vi "Approach then IT.vi"(7 "Computer called (T/F)":bool) -> ()   [LabVIEW 2023]
uses:
  Sub_Vi/TypeDefsControls/Zposition.ctl
  Sub_Vi/TypeDefsControls/Piezo Velocity.ctl
  Sub_Vi/TypeDefsControls/Voltage.ctl
  Sub_Vi/TypeDefsControls/Xposition.ctl
  Sub_Vi/TypeDefsControls/Yposition.ctl
  Sub_Vi/TypeDefsControls/Time.ctl
  Sub_Vi/TypeDefs/WayPointCluster.ctl
  Sub_Vi/TypeDefs/ChangeOnFly.ctl
  Sub_Vi/TypeDefs/Display.ctl
  Sub_Vi/TypeDefs/Settings.ctl
  Sub_Vi/TypeDefsControls/Feedback Type.ctl
  Settings.vi
panel:
  in  "Tab Control 2":T1(tab)
  out "C1":dbl[](graph)
  out "C2":dbl[](graph)
  out "C3":dbl[](graph)
  in  "Feedback Type":T2=enum."Current 1"
  in  "Tab Control":enum32{"C1 vs Z", "C2 vs Z", "C3 vs Z"}(tab)
  out "Z vs C1":cluster{"Y":dbl[], "Y":dbl[]}[](graph)
  out "Z vs C2":cluster{"Y":dbl[], "Y":dbl[]}[](graph)
  out "Z vs C3":cluster{"Y":dbl[], "Y":dbl[]}[](graph)
  in  "SettingsCluster":T3={"Sample Rate (us)"=1, "Samples Per Data Point (int, power of 2)"=1000, "DistanceToBulk (um)"=-1.0, "HoldTimeScaler"=1, "SaveData"=TRUE, "DistanceToBulk (um) 2"=-1.0, "DistanceToBulk (um) 3"=-1.0}
  in  "Display Cluster":T4
  in  "ChangeonFly":T5
  in  "WayPointCluster":T6
  in  "IT Time (s)":T7=8.0 min=0.0
  in  "Start scan Button":bool
  in  "Stop":bool
  in  "Pause":bool
  in  "IT Voltage (V)":T8 min=-10.0 max=10.0
  in  "Greater Than":bool=TRUE
  in  "Set X":bool
  in  "Set Y":bool
  in  "Y":T9=50.0 min=0.0 max=100000.0
  in  "X":T10=50.0 min=0.0 max=100000.0
  in  "Retract after approach":bool=TRUE
  in  "Approach Voltage (V)":T8=0.35 min=-10.0 max=10.0
  in  "Approach Rate (µm/s)":T11=0.1 min=0.0
  in  "End Extension (µm)":T12 min=0.0 max=100000.0
  in  "Start Extention (µm)":T12=150.0 min=0.0 max=100000.0
  in  "Feedback Threshold (A)":dbl
  in  "Start Scanning Button":bool
  out "Lockin Phase":dbl[](graph)
  out "Lockin Amp":dbl[](graph)
  # "Settings"
  # "Pause at"
  # "Advanced Settings"
  # "IT Controls"
  # "Voltage Profile"
  # "Approach"
  # "Retract"
  # "IT"
  # "IT\nVoltage"
  # "Approach\nVoltage"
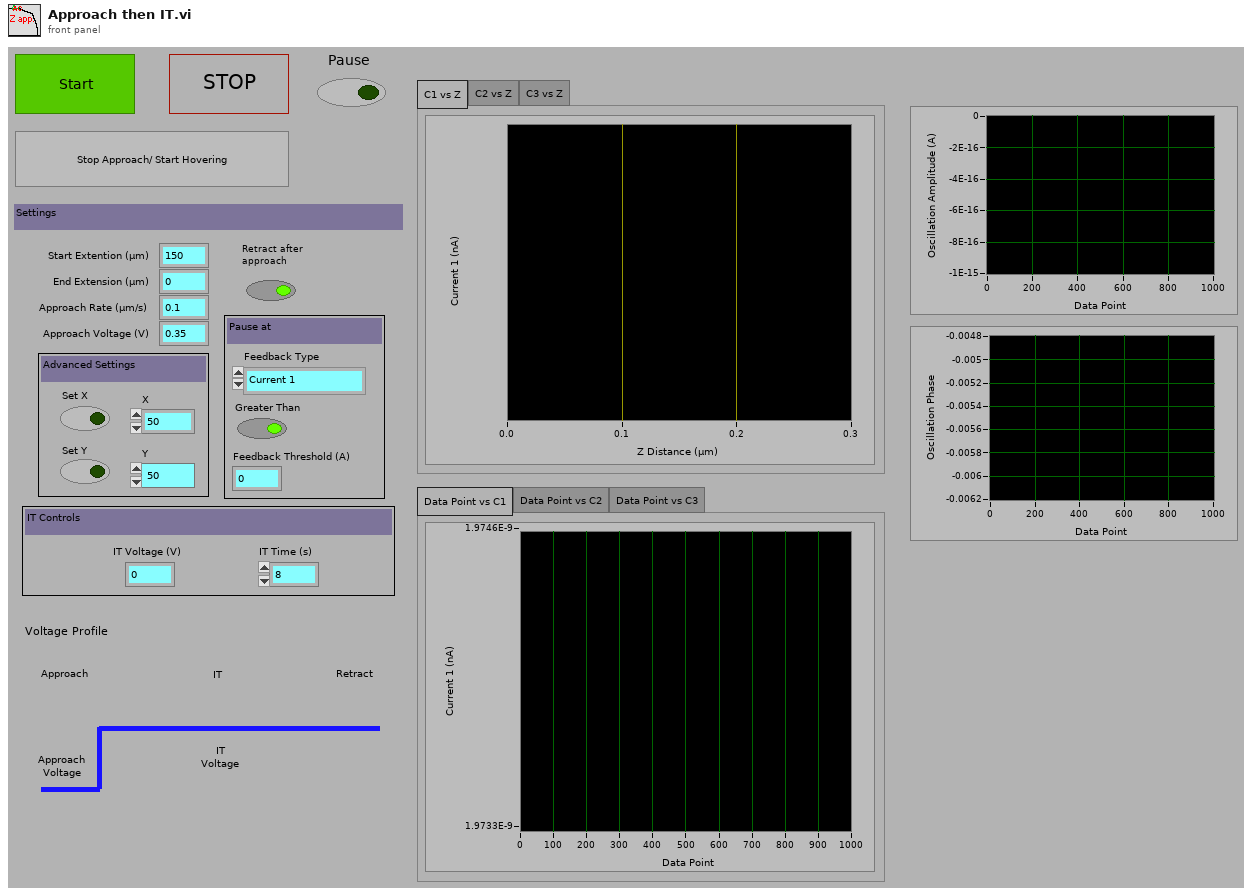
[diagram p1: front panel]
types:
  T1 = enum32{"Data Point vs C1", "Data Point vs C2", "Data Point vs C3"}
  T2 = typedef "Feedback Type.ctl" = enum16{"AC Magnitude", "Current 1", "Current 2", "Phase"}
  T3 = typedef "Settings.ctl" = cluster{"Sample Rate (us)":u32, "Samples Per Data Point (int, power of 2)":i16, "DistanceToBulk (um)":dbl, "HoldTimeScaler":u64, "SaveData":bool, "DistanceToBulk (um) 2":dbl, "DistanceToBulk (um) 3":dbl}
  T4 = typedef "Display.ctl" = cluster{"X":refnum<vi>, "Y":refnum<vi>, "Z":refnum<vi>, "Amp":refnum<vi>, "Phase":refnum<vi>, "t vs Z":refnum<vi>, "t vs C1":refnum<vi>, "t vs C2":refnum<vi>, "t vs C3":refnum<vi>, "t vs Amp":refnum<vi>, "t vs Phase":refnum<vi>, "t vs X":refnum<vi>, "t vs Y":refnum<vi>, "Z vs C1":refnum<vi>, "Z vs C2":refnum<vi>, "Z vs C3":refnum<vi>, "V vs C1":refnum<vi>, "V vs C2":refnum<vi>, "V vs C3":refnum<vi>, "X/Y/Z F":refnum<vi>, "X/Y/Z R":refnum<vi>, "X/Y/C1 F":refnum<vi>, "X/Y/C1 R":refnum<vi>, "X/Y/C2 F":refnum<vi>, "X/Y/C2 R":refnum<vi>, "X/Y/C3 F":refnum<vi>, "X/Y/C3 R":refnum<vi>, "NumberOfLines":u16, "um Per Pixel":dbl, "um Per Line":dbl, "X Center":dbl, "Hop X/Y/Z":refnum<vi>, "Hop X/Y/C1":refnum<vi>, "Hop X/Y/C2":refnum<vi>, "Hop X/Y/C3":refnum<vi>, "X Width":dbl, "Y Width":dbl, "Hopping Distance":dbl, "V2 vs C1":refnum<vi>, "V vs Phase":refnum<vi>, "Y Center":dbl, "Number of Pixels":dbl, "V2 vs C2":refnum<vi>, "V2 vs C3":refnum<vi>, "V vs y":refnum<vi>, "V2 vs y":refnum<vi>, "Z vs Amp":refnum<vi>, "Z vs Phase":refnum<vi>}
  T5 = typedef "ChangeOnFly.ctl" = cluster{"Stop (boolean)":refnum<vi>, "Pause (boolean)":refnum<vi>, "EndCurrentLine (boolean)":refnum<vi>, "max movement per update step (Interger, nm)":refnum<vi>, "P (float, arb)":refnum<vi>, "Feedback set point (double, Amps)":refnum<vi>, "Voltage (double, V)":refnum<vi>, "Feedback set point 2 (double, Amps)":refnum<vi>, "Stop on Greater Than 2? (boolean)":refnum<vi>, "Stop on Greater Than? (boolean)":refnum<vi>, "Voltage 2 (double, V)":refnum<vi>, "Feedback Type (enum)":refnum<vi>, "Feedback Type 2 (enum)":refnum<vi>}
  T6 = typedef "WayPointCluster.ctl" = cluster{"X (um)":dbl[], "Y (um)":dbl[], "Z (um)":dbl[], "V (V)":dbl[], "X Velocity (um s-1)":dbl[], "Y Velocity (um s-1)":dbl[], "Z Velocity (um s-1)":dbl[], "V Velocity (V s-1)":dbl[], "FeedBack Type (enum)":u16[], "Move X (boolean)":bool[], "Move Y (boolean)":bool[], "Move Z (boolean)":bool[], "Move V (boolean)":bool[], "Jump V (boolean)":bool[], "Hold (boolean)":bool[], "Hold Time":u32[], "V2 (V)":dbl[], "Move V2":bool[], "V2 Velocity (V s-1)":dbl[], "Jump V2 (boolean)":bool[], "Update z Position delta (ms)":i16[], "Hold Feedback1":bool[], "Move Z PicoMotor":bool[], " Z PicoMotor Direction":bool[], "DIO0":bool[]}
  T7 = typedef "Time.ctl" = dbl
  T8 = typedef "Voltage.ctl" = dbl
  T9 = typedef "Yposition.ctl" = dbl
  T10 = typedef "Xposition.ctl" = dbl
  T11 = typedef "Piezo Velocity.ctl" = dbl
  T12 = typedef "Zposition.ctl" = dbl
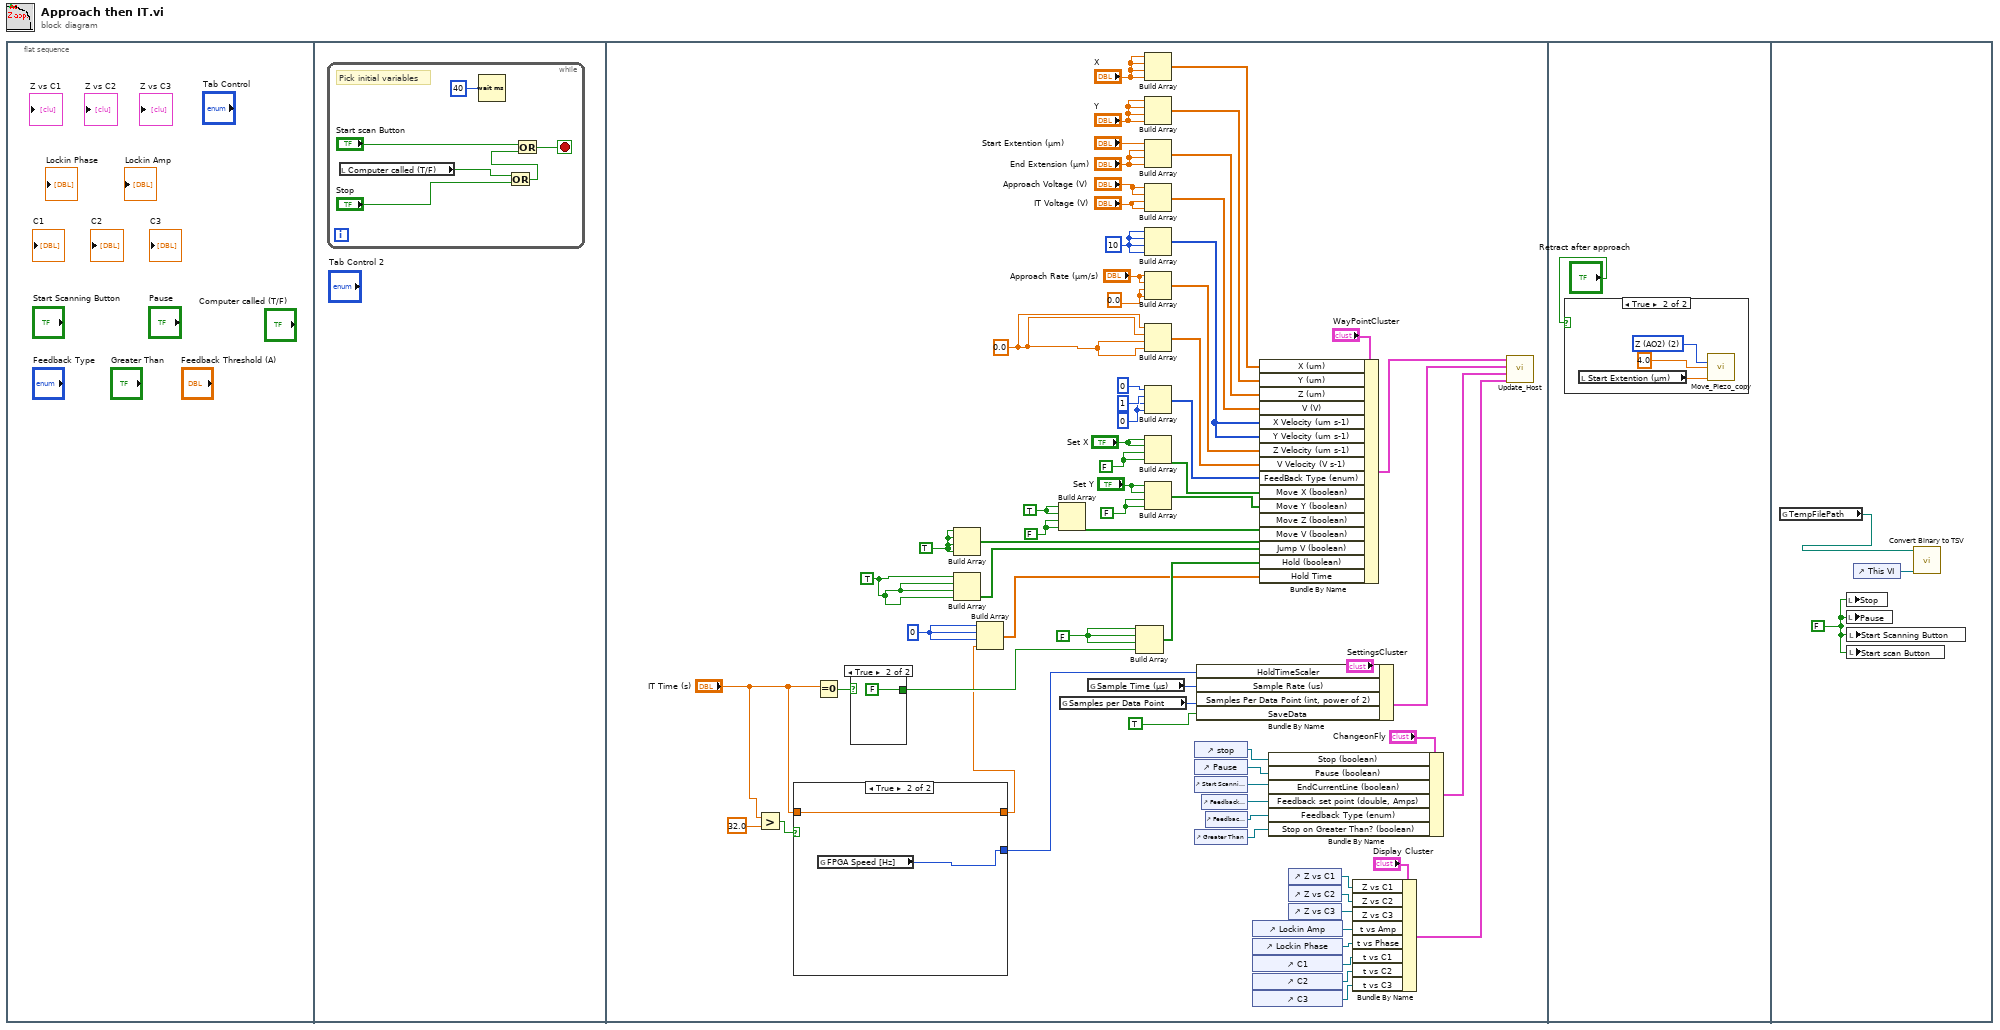
[diagram p0: block diagram]
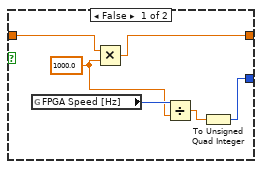
[diagram p2: hidden frame]
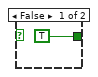
[diagram p3: hidden frame]
diagram:
  n1 = flat-sequence {
    frame #0 {
    }
    frame #1 {
      n2 = while {
        stop <- w6 stop-if-true
        # "Pick initial variables"
        n3 = local read "Computer called (T/F)"() -> (w1:bool)
        n4 = Wait (ms)(milliseconds to wait=u32 40) -> ()  [unwired: 1 out]
        n5 = Or(x=w1, y="Stop") -> (x .or. y?=w2:bool)
        n6 = Or(x="Start scan Button", y=w2) -> (x .or. y?=w6:bool)
      }
    }
    frame #2 {
      w52 = u32 0 ("element")
      w15 = TRUE ("Set Z")
      w20 = TRUE ("element")
      w53 = FALSE ("element")
      w56 = FALSE ("element")
      w57 = FALSE ("element")
      w8 = u16 0 ("element")
      w14 = 0.0
      w26 = 0.0 ("element")
      w17 = FALSE ("Set Z")
      w62 = TRUE ("Set Z")
      w55 = 10
      n7 = Greater?(x="IT Time (s)", y=T7 32.0) -> (0:w12:bool)
      n8 = case shown="True" w12 {
        tunnel: "IT Time (s)" -> [w82 w84]
        tunnel: [w81 w84] -> w10
        tunnel: [w77 w83] -> w9
        frame False {
          w79 = 1000.0 ("y")
          n9 = global read "Settings.vi" "FPGA Speed [Hz]"() -> (w80:i64)
          n10 = Multiply(x=w82, y=w79) -> (x*y=w81:T7)
          n11 = Divide(x=w80, y=w79) -> (x/y=w78:dbl)
          n12 = To Unsigned Quad Integer(1:w78) -> (0:w77:u64)
        }
        frame True {
          n13 = global read "Settings.vi" "FPGA Speed [Hz]"() -> (w83:i64)
        }
      }
      n14 = Equal To 0?(x="IT Time (s)") -> (x = 0?=w51:bool)
      n15 = case shown="True" w51 {
        tunnel: [TRUE ("Set Z") FALSE ("Set Z")] -> w16
        frame False {
        }
        frame True {
        }
      }
      n16 = Build Array(w20, w20, w20, w20) -> (w21:bool[])
      n17 = Build Array(w15, w15, w15, w15) -> (w67:bool[])
      n18 = Build Array(w52, w52, w52, w10) -> (w65:T7[])
      n19 = Build Array(w62, w62, w53, w53) -> (w54:bool[])
      n20 = global read "Settings.vi" "Samples per Data Point"() -> (w60:u16)
      n21 = global read "Settings.vi" "Sample Time (µs)"() -> (w61:u32)
      n22 = Build Array(w17, w17, w17, w16) -> (w70:bool[])
      n23 = Build Array("X", "X", "X", "X") -> (w75:T10[])
      n24 = Build Array("Y", "Y", "Y", "Y") -> (w74:T9[])
      n25 = Build Array("Start Extention (µm)", "End Extension (µm)", "End Extension (µm)", "End Extension (µm)") -> (w18:T12[])
      n26 = Build Array("Approach Voltage (V)", "Approach Voltage (V)", "IT Voltage (V)", "IT Voltage (V)") -> (w58:T8[])
      n27 = Build Array(w55, w55, w55, w55) -> (w76:i32[])
      n28 = Build Array("Approach Rate (µm/s)", "Approach Rate (µm/s)", w26, w26) -> (w73:T11[])
      n29 = Build Array(w14, w14, w14, w14) -> (w69:dbl[])
      n30 = Build Array(u16 0 ("element"), u16 1, w8, w8) -> (w68:u16[])
      n31 = Build Array("Set X", "Set X", w56, w56) -> (w72:bool[])
      n32 = Build Array("Set Y", "Set Y", w57, w57) -> (w19:bool[])
      n33 = control-ref of="stop"() -> (w35:refnum<vi>)
      n34 = control-ref of="Pause"() -> (w36:refnum<vi>)
      n35 = control-ref of="Start Scanning Button"() -> (w37:refnum<vi>)
      n36 = control-ref of="Greater Than"() -> (w39:refnum<vi>)
      n37 = Bundle By Name(cluster="SettingsCluster", "HoldTimeScaler"=w9, "Sample Rate (us)"=w61, "Samples Per Data Point (int, power of 2)"=w60, "SaveData"=TRUE) -> (w71:T3)
      n38 = control-ref of="Feedback Threshold (A)"() -> (w40:refnum<vi>)
      n39 = control-ref of="Feedback Type"() -> (w38:refnum<vi>)
      n40 = control-ref of="Lockin Amp"() -> (w49:refnum<vi>)
      n41 = control-ref of="Lockin Phase"() -> (w48:refnum<vi>)
      n42 = control-ref of="C1"() -> (w45:refnum<vi>)
      n43 = control-ref of="C2"() -> (w44:refnum<vi>)
      n44 = control-ref of="C3"() -> (w43:refnum<vi>)
      n45 = Bundle By Name(cluster="WayPointCluster", "X (um)"=w75, "Y (um)"=w74, "Z (um)"=w18, "V (V)"=w58, "X Velocity (um s-1)"=w76, "Y Velocity (um s-1)"=w76, "Z Velocity (um s-1)"=w73, "V Velocity (V s-1)"=w69, "FeedBack Type (enum)"=w68, "Move X (boolean)"=w72, "Move Y (boolean)"=w19, "Move Z (boolean)"=w54, "Move V (boolean)"=w21, "Jump V (boolean)"=w67, "Hold (boolean)"=w70, "Hold Time"=w65) -> (w33:T6)
      n46 = Bundle By Name(cluster="ChangeonFly", "Stop (boolean)"=w35, "Pause (boolean)"=w36, "EndCurrentLine (boolean)"=w37, "Feedback set point (double, Amps)"=w40, "Feedback Type (enum)"=w38, "Stop on Greater Than? (boolean)"=w39) -> (w41:T5)
      n47 = control-ref of="Z vs C1"() -> (w64:refnum<vi>)
      n48 = control-ref of="Z vs C2"() -> (w47:refnum<vi>)
      n49 = control-ref of="Z vs C3"() -> (w46:refnum<vi>)
      n50 = Bundle By Name(cluster="Display Cluster", "Z vs C1"=w64, "Z vs C2"=w47, "Z vs C3"=w46, "t vs Amp"=w49, "t vs Phase"=w48, "t vs C1"=w45, "t vs C2"=w44, "t vs C3"=w43) -> (w32:T4)
      n51 = call "Update_Host.vi"("Display Cluster"=w32, "ChangeonFly"=w41, "SettingsCluster"=w71, "WayPointCluster"=w33) -> ()  [unwired: 6 in]
    }
    frame #3 {
      n52 = case shown="True" "Retract after approach" {
        frame False {
        }
        frame True {
          w90 = u16 2 items=["X (AO0)", "Y (AO1)", "Z (AO2)", "V (AO3)"] ("Channel")
          n53 = local read "Start Extention (µm)"() -> (w88:T12)
          n54 = call "Move_Piezo_copy.vi"("Piezo"=w90, "Movement Speed (µm/s)"=4.0 ("Scan Rate (um/s)"), "Position (µm) (or V)"=w88) -> ()  [unwired: 13 in]
        }
      }
    }
    frame #4 {
      w92 = FALSE ("stop recording")
      n55 = global read "Settings.vi" "TempFilePath"() -> (w91:path)
      n56 = local write "Stop"(w92) -> ()
      n57 = local write "Pause"(w92) -> ()
      n58 = local write "Start Scanning Button"(w92) -> ()
      n59 = local write "Start scan Button"(w92) -> ()
      n60 = control-ref of="This VI"() -> (w93:refnum<vi>)
      n61 = call "Convert Binary to TSV.vi"("This VI"=w93, "TDMS DataFile Name"=w91) -> ()  [unwired: 10 in]
    }
  }
